vi "Top Level VI Reference.vi"() -> (0 "Top Level VI Reference":refnum<vi>)   [LabVIEW 2012, in "VIRef.lvlib"]
uses:
  VIRef.lvlib
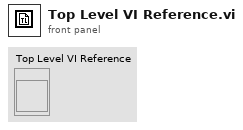
[diagram p1: front panel]
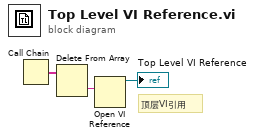
[diagram p0: block diagram]
diagram:
  # "顶层VI引用"
  n1 = Call Chain() -> (call chain=w3:string[])
  n2 = Delete From Array(array=w3) -> (deleted portion=w2:string)  [unwired: 2 in, 1 out]
  n3 = Open VI Reference(vi path=w2) -> (vi reference=→"Top Level VI Reference":refnum<vi>)  [unwired: 5 in, 1 out]
